vi "Read Conversion Time.vi"(8 "error in":errorcluster, 11 "thermocouple mode in":refnum<class "Thermocouple Mode.lvclass">) -> (0 "error out":errorcluster, 2 "conversion time":T1, 3 "thermocouple mode out":refnum<class "Thermocouple Mode.lvclass">)   [LabVIEW 2017, in "Scan Engine Scripting.lvlib" / "Thermocouple Mode.lvclass"]
uses:
  Thermocouple Mode.lvclass
  Conversion Time.ctl
  Thermocouple Mode.lvclass/Thermocouple Mode.ctl
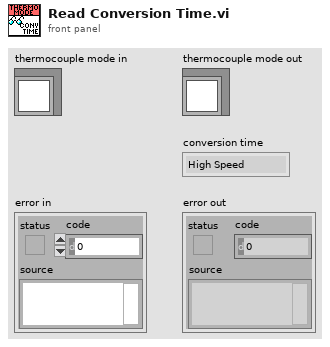
[diagram p1: front panel]
types:
  T1 = typedef "Scan Engine Scripting.lvlib/Thermocouple Mode.lvclass/Conversion Time.ctl" = enum16{"High Speed", "High Resolution"}
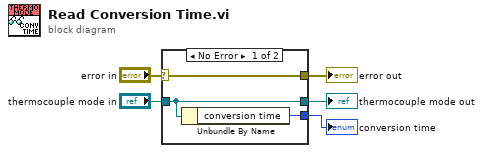
[diagram p0: block diagram]
diagram:
  n1 = case shown="No Error" "error in" {
    selector: "error in" -> [w8 w9]
    tunnel: [w8 w9] -> w4
    tunnel: [w7 w10] -> w2
    tunnel: "thermocouple mode in" -> [w7 w10]
    tunnel: [w6 _] -> w1
    frame No Error {
      n2 = Unbundle By Name(w7) -> ("conversion time"=w6:T1)
    }
    frame Error {
    }
  }
  "error out" <- w4
  "thermocouple mode out" <- w2
  "conversion time" <- w1
